vi "Parker Stepper Test.vi"() -> ()   [LabVIEW 2021]
panel:
  in  "Time between steps (S)":dbl=1.0 format="%.2f"
  in  "stop":bool
  in  "Parameters":dbl[](array[numeric]) format="%.2f"
  out "Data Out":dbl[](array[numeric]) format="%.2f"
  in  "Instrument Address":refnum<visa-resource-name>
  in  "Init":bool
  # "Motor Number"
  # "Step Size"
  # "Final Position"
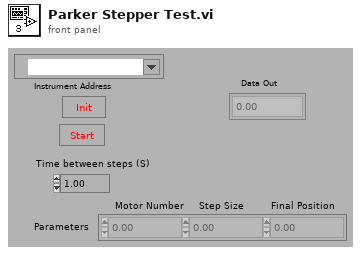
[diagram p1: front panel]
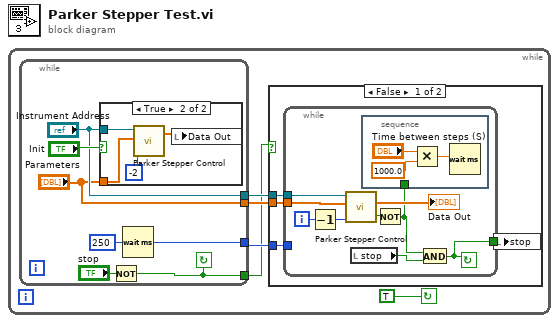
[diagram p0: block diagram]
diagram:
  n1 = while {
    stop <- TRUE continue-if-true
    n2 = while {
      tunnel: ["Parameters"] -> w4
      tunnel: ["Instrument Address"] -> w3
      tunnel: [w9] -> w2
      tunnel: [w6] -> w1
      stop <- w6 continue-if-true
      n3 = case shown="True" "Init" {
        tunnel: "Instrument Address" -> [_ w16]
        tunnel: "Parameters" -> [_ w15]
        frame False {
        }
        frame True {
          n4 = call "Parker Stepper Control.vi"("Point #"=-2, "Parameters"=w15, "Instrument Address"=w16) -> ("Data Out"=w13:dbl[])  [unwired: 1 in, 1 out]
          n5 = local write "Data Out"(w13) -> ()
        }
      }
      n6 = Not(x="stop") -> (.not. x?=w6:bool)
      n7 = Wait (ms)(milliseconds to wait=u32 250) -> (millisecond timer value=w9:u32)
    }
    n8 = case shown="False" w1 {
      tunnel: w2 -> [w20 _]
      tunnel: w3 -> [w19 _]
      tunnel: w4 -> [w18 _]
      frame False {
        n9 = while {
          tunnel: [w23] -> w17
          tunnel: w20 -> [_]
          tunnel: w19 -> [w24]
          tunnel: w18 -> [w26]
          i -> [w27]
          stop <- w23 continue-if-true
          n10 = Decrement(x=w27) -> (x-1=w21:i32)
          n11 = call "Parker Stepper Control.vi"("Point #"=w21, "Parameters"=w26, "Instrument Address"=w24) -> ("Stop"=w25:bool, "Data Out"=→"Data Out":dbl[])  [unwired: 1 in]
          n12 = local read "stop"() -> (w29:bool)
          n13 = Not(x=w25) -> (.not. x?=w22:bool)
          n14 = stacked-sequence {
            tunnel: w22 -> [_]
            frame #0 {
              n15 = Multiply(x="Time between steps (S)", y=1000.0) -> (x*y=w32:dbl)
              n16 = Wait (ms)(milliseconds to wait=w32) -> ()  [unwired: 1 out]
            }
          }
          n17 = And(x=w22, y=w29) -> (x .and. y?=w23:bool)
        }
        n18 = local write "stop"(w17) -> ()
      }
      frame True {
      }
    }
  }
